vi "Data_SetStreamInfo.vi"(8 "error in (no error)":errorcluster, 9 "block":i32, 10 "streamId":string, 11 "data in":variant) -> (0 "error out":errorcluster, 3 "data out":variant)   [LabVIEW 2017, in "FileManager.lvlib"]
uses:
  <vilib>/addons/InsightCM/Devices/Shared/Common/FileManager/FileManager.lvlib
  <vilib>/addons/InsightCM/Devices/Shared/Common/FileManager/controls/DataPropertyNames.ctl
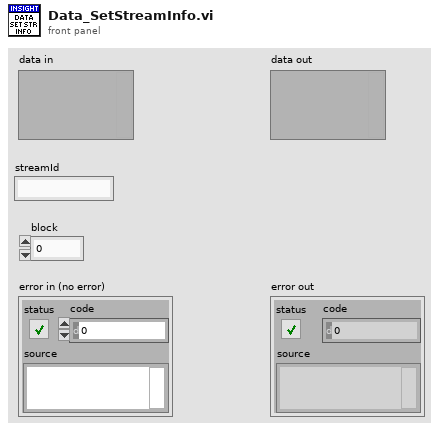
[diagram p1: front panel]
types:
  T1 = typedef "DataPropertyNames.ctl" = enum16{"Type", "EventRef", "FilePath", "DataGroup", "AcquisitionTimestamp", "StreamId", "StreamBlock", "TrendPointsOnly", "ExtraLargeFile"}
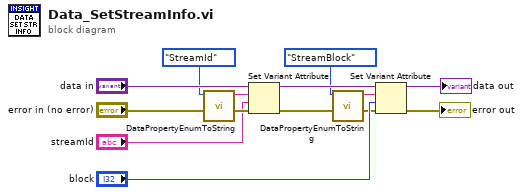
[diagram p0: block diagram]
diagram:
  n1 = call <vilib>:"DataPropertyEnumToString.vi"("property"=DataPropertyNames."StreamId" ("Names")) -> ("string"=w3:string)  [unwired: 10 in]
  n2 = Set Variant Attribute(Variant="data in", name=w3, value="streamId", error in="error in (no error)") -> (Variant out=w5:variant, error out=w6:errorcluster)  [unwired: 1 out]
  n3 = call <vilib>:"DataPropertyEnumToString.vi"("property"=DataPropertyNames."StreamBlock" ("Names")) -> ("string"=w1:string)  [unwired: 10 in]
  n4 = Set Variant Attribute(Variant=w5, name=w1, value="block", error in=w6) -> (Variant out=→"data out":variant, error out=→"error out":errorcluster)  [unwired: 1 out]
